vi "Main.vi"(7 "sweep rate, /min":dbl=0.2, 8 "sweep to:":dbl=-0.5, 9 "sweep":T6(radio)=enum."time_sweep") -> ()   [LabVIEW 2017] (continued)
                        n2125 = property on="data_caption" class="Str"() -> ("Value"=w2775:string)  [unwired: 2 in, 2 out]
                        n2126 = local read "Data file:"() -> (w2776:path)
                        n2127 = Concatenate Strings(w2775, "\r") -> (w2777:string)
                        n2128 = Write to Text File(file (use dialog)=w2776, text=w2777) -> ()  [unwired: 2 in, 3 out]
                      }
                      frame True {
                        # "records the fist line into the both upa nd down data file\nwhen table index=0"
                        n2129 = property on="Table Index" class="DigNum (strict)"() -> ("Value"=w2779:dbl)  [unwired: 2 in, 2 out]
                        n2130 = Equal To 0?(x=w2779) -> (x = 0?=w2778:bool)
                        n2131 = case shown="True" w2778 {
                          frame False {
                          }
                          frame True {
                            n2132 = property on="data_caption" class="Str"() -> ("Value"=w2783:string)  [unwired: 2 in, 2 out]
                            n2133 = local read "Data file:"() -> (w2780:path)
                            n2134 = Concatenate Strings(w2783, "\r") -> (w2782:string)
                            n2135 = Write to Text File(file (use dialog)=w2780, text=w2782) -> ()  [unwired: 2 in, 3 out]
                          }
                        }
                      }
                    }
                  }
                  frame True {
                    # "records the fist line into the both upa nd down data file\nwhen table index=0"
                    n2136 = property on="Table Index" class="DigNum (strict)"() -> ("Value"=w2787:dbl)  [unwired: 2 in, 2 out]
                    n2137 = property on="HyperLoop Index" class="DigNum (strict)"() -> ("Value"=w2788:dbl)  [unwired: 2 in, 2 out]
                    n2138 = Equal To 0?(x=w2787) -> (x = 0?=w2785:bool)
                    n2139 = Equal To 0?(x=w2788) -> (x = 0?=w2786:bool)
                    n2140 = And(x=w2786, y=w2785) -> (x .and. y?=w2784:bool)
                    n2141 = case shown="True" w2784 {
                      frame False {
                      }
                      frame True {
                        n2142 = property on="data_caption" class="Str"() -> ("Value"=w2792:string)  [unwired: 2 in, 2 out]
                        n2143 = local read "Data file:"() -> (w2789:path)
                        n2144 = Concatenate Strings(w2792, "\r") -> (w2791:string)
                        n2145 = Write to Text File(file (use dialog)=w2789, text=w2791) -> ()  [unwired: 2 in, 3 out]
                      }
                    }
                  }
                }
              }
            }
            n2146 = property on="Figure_axis" class="Arr (strict)"() -> ("Value"=w2759:string[])  [unwired: 2 in, 2 out]
            n2147 = property on="Xaxis" class="Ring (strict)"("Strings []"=w2759) -> ()  [unwired: 2 in, 2 out]
            n2148 = property on="Stop Sweep" class="Bool"("DisabledEnum"=T12."Enabled" ("Disabled")) -> ()  [unwired: 2 in, 2 out]
            n2149 = property on="Yright" class="Ring (strict)"("Strings []"=w2759) -> ()  [unwired: 2 in, 2 out]
            n2150 = property on="Yaxis" class="Ring (strict)"("Strings []"=w2759) -> ()  [unwired: 2 in, 2 out]
          }
        }
        n2151 = call "timeInSeconds.vi"() -> ("Numeric"=w1798:dbl)  [unwired: 2 in, 1 out]
        n2152 = while {
          shift-right: [w2844] -> _
          shift-left: w1797 -> [w2845]
          shift-right: [w2842] -> w1796
          shift-left: w1794 -> [w2841]
          tunnel: w1798 -> [w2839]
          stop <- w2832 stop-if-true
          # "initial value"
          # "Measure the selected channels"
          # "data array"
          # "this loop stops when target value is reached"
          # "error cluster to determine data flow"
          n2153 = stacked-sequence {
            tunnel: [_ _ w2866 _ _ _] -> w2833
            tunnel: [_ _ w2865 _ _ _] -> w2843
            tunnel: w2841 -> [_ _ w2859 _ _ _]
            tunnel: [w2851 _ _ _ _ _] -> w2840
            tunnel: w2839 -> [_ _ _ w2889 _ _]
            tunnel: [_ _ w2859 _ _ _] -> w2835
            tunnel: [_ _ _ _ _ w3552] -> w2831
            frame #0 {
              # "time is measured at the beginning\nand at the end of the cycle to\ncalculate delay time required to\nkeep set sweep rate"
              n2154 = flat-sequence {
                tunnel: [w2853] -> w2851
                frame #0 {
                  n2155 = property on="time delay, ms" class="DigNum (strict)"() -> ("Value"=w2852:dbl)  [unwired: 2 in, 2 out]
                  n2156 = Wait (ms)(milliseconds to wait=w2852) -> ()  [unwired: 1 out]
                }
                frame #1 {
                  n2157 = Tick Count (ms)() -> (millisecond timer value=w2853:u32)
                }
              }
            }
            frame #1 {
              w2854 = dbl[] []  # Empty array for data
              # "clear data array before each measurement cycle"
              n2158 = property on="data" class="Arr (strict)"("Value"=w2854) -> ()  [unwired: 2 in, 2 out]
            }
            frame #2 {
              # "add next sweep value to the data array"
              n2159 = property on="data" class="Arr (strict)"() -> ("Value"=w2864:dbl[])  [unwired: 2 in, 2 out]
              n2160 = property on="Sweep B" class="Bool (strict)"() -> ("Value"=w2856:bool)  [unwired: 2 in, 2 out]
              n2161 = local read "sweep"() -> (w2862:T6)
              n2162 = Not(x=w2856) -> (.not. x?=w2855:bool)
              n2163 = Equal?(x=w2862, y=T19."Radio Selection 7" ("sweep")) -> (x = y?=w2858:bool)
              n2164 = And(x=w2858, y=w2855) -> (x .and. y?=w2857:bool)
              n2165 = case shown="False" w2857 {
                tunnel: [w2873 w2885] -> w2866
                tunnel: [w2867 w2884] -> w2865
                tunnel: w2859 -> [_ w2882]
                tunnel: [w2867 w2882] -> w2860
                frame True {
                  n2166 = disable-structure shown="Disabled" {
                    disable-tunnel: [w2876 _] -> _
                    disable-tunnel: [w2875 _] -> _
                    frame Disabled {
                      n2167 = stacked-sequence {
                        tunnel: [_ w2878 _] -> w2876
                        tunnel: [_ _ w2880] -> w2875
                        frame #0 {
                          n2168 = local read "Hulk_SMS_addr"() -> (w2877:refnum<visa-resource-name>)
                          n2169 = VISA Clear(VISA resource name=w2877) -> ()  [unwired: 1 in, 2 out]
                        }
                        frame #1 {
                          # "acquires current output value"
                          n2170 = local read "Hulk_SMS_addr"() -> (w2879:refnum<visa-resource-name>)
                          n2171 = call "SMS_GET_OUTPUT.vi"("Hulk_SMS_addr"=w2879) -> ("Numeric"=w2878:dbl)  [unwired: 1 in, 2 out]
                        }
                        frame #2 {
                          # "checks, wheter ramp was finished"
                          n2172 = local read "Hulk_SMS_addr"() -> (w2881:refnum<visa-resource-name>)
                          n2173 = call "SMS_RAMP_STATUS.vi"("Hulk_SMS_addr"=w2881) -> ("selection"=w2880:bool)  [unwired: 1 in, 2 out]
                        }
                      }
                    }
                    frame Enabled {
                    }
                  }
                  n2174 = property on="iPS_addr_sweep" class="VISAName"() -> ("Value"=w2869:refnum<visa-resource-name>)  [unwired: 2 in, 2 out]
                  n2175 = property on="sweep to:" class="DigNum (strict)"() -> ("Value"=w2874:dbl)  [unwired: 2 in, 2 out]
                  n2176 = call "iPSread.vi"("iPSreadCtrl"=iPSreadCtrl."MagnetField", "VISA resource name"=w2869) -> ("number"=w2867:dbl)  [unwired: 6 in, 3 out]
                  n2177 = property on="Tolerance_Sweep" class="DigNum (strict)"() -> ("Value"=w2870:dbl)  [unwired: 2 in, 2 out]
                  n2178 = Subtract(x=w2867, y=w2874) -> (x-y=w2872:dbl)
                  n2179 = Absolute Value(x=w2872) -> (abs(x)=w2871:dbl)
                  n2180 = Less Or Equal?(x=w2871, y=w2870) -> (x <= y?=w2873:bool)
                }
                frame False {
                  # "calculate next value"
                  n2181 = call "CalculateNextValue.vi"("Target a 2"="sweep to:", "Channel a source value"=w2882, "Ch a sweep rate units/min"="sweep rate, /min", "time between points, sec"="time/point, sec", "Source a"=Source."Voltage") -> ("Target a"=w2884:dbl, "Boolean"=w2885:bool)
                }
              }
              n2182 = Build Array (concatenate)(w2864, w2860) -> (w2863:dbl[])
              n2183 = property on="data" class="Arr (strict)"("Value"=w2863) -> ()  [unwired: 2 in, 2 out]
            }
            frame #3 {
              n2184 = stacked-sequence "measurement sequence" {
                tunnel: w2889 -> [_ _ _ _ _ _ _ _ _ _ _ _ _ _ _ _ _ _ _ _ _ _ _ _ _ _ _ _ _ _ _ _ _ _ _ _ _ _ w3427 _ _ _ _ _ _ _ _ _ _ _ _ _]
                frame #0 {
                  # "check if in-phase\nsignal on lock-in 1 \nis to be measured"
                  n2185 = property on="data" class="Arr (strict)"() -> ("Value"=w2891:dbl[])  [unwired: 2 in, 2 out]
                  n2186 = local read "SR830 1 ip"() -> (w2890:bool)
                  n2187 = case shown="True" w2890 {
                    tunnel: w2891 -> [w2893 w2902]
                    tunnel: [w2893 w2901] -> w2892
                    frame False {
                      # "we are not measuring in phase signal on lock-in 1 (SR830_1_ip)"
                    }
                    frame True {
                      # "we are  measuring lock-in 1, in phase (SR830_1_ip)"
                      n2188 = local read "SR830 1 addr"() -> (w2895:u8)
                      n2189 = Number To Decimal String(number=w2895) -> (decimal integer string=w2894:string)  [unwired: 1 in]
                      n2190 = GPIB Write(0:w2894, 1:"OUTR?1") -> (6:w2900:errorcluster)  [unwired: 3 in, 1 out]
                      n2191 = GPIB Read(0:w2894, 1:3200, 3:w2900) -> (5:w2898:string)  [unwired: 2 in, 2 out]
                      n2192 = Fract/Exp String To Number(string=w2898) -> (number=w2897:dbl)  [unwired: 3 in, 1 out]
                      n2193 = Build Array (concatenate)(w2902, w2897) -> (w2901:dbl[])
                    }
                  }
                  n2194 = property on="data" class="Arr (strict)"("Value"=w2892) -> ()  [unwired: 2 in, 2 out]
                }
                frame #1 {
                  # "check if out-of-phase\nsignal on lock-in 1 \nis to be measured"
                  n2195 = property on="data" class="Arr (strict)"() -> ("Value"=w2904:dbl[])  [unwired: 2 in, 2 out]
                  n2196 = local read "SR830 1 oop"() -> (w2903:bool)
                  n2197 = case shown="True" w2903 {
                    tunnel: w2904 -> [w2906 w2915]
                    tunnel: [w2906 w2914] -> w2905
                    frame False {
                      # "we are not measuring out of phase signal on lock-in 1 (SR830_1_oop)"
                    }
                    frame True {
                      # "we are  measuring lock-in 1, out of phase (SR830_1_oop)"
                      n2198 = local read "SR830 1 addr"() -> (w2908:u8)
                      n2199 = Number To Decimal String(number=w2908) -> (decimal integer string=w2907:string)  [unwired: 1 in]
                      n2200 = GPIB Write(0:w2907, 1:"OUTR?2") -> (6:w2913:errorcluster)  [unwired: 3 in, 1 out]
                      n2201 = GPIB Read(0:w2907, 1:3200, 3:w2913) -> (5:w2911:string)  [unwired: 2 in, 2 out]
                      n2202 = Fract/Exp String To Number(string=w2911) -> (number=w2910:dbl)  [unwired: 3 in, 1 out]
                      n2203 = Build Array (concatenate)(w2915, w2910) -> (w2914:dbl[])
                    }
                  }
                  n2204 = property on="data" class="Arr (strict)"("Value"=w2905) -> ()  [unwired: 2 in, 2 out]
                }
                frame #2 {
                  # "check if in-phase\nsignal on lock-in 2 \nis to be measured"
                  n2205 = property on="data" class="Arr (strict)"() -> ("Value"=w2917:dbl[])  [unwired: 2 in, 2 out]
                  n2206 = local read "SR830 2 ip"() -> (w2916:bool)
                  n2207 = case shown="True" w2916 {
                    tunnel: w2917 -> [w2919 w2928]
                    tunnel: [w2919 w2927] -> w2918
                    frame False {
                      # "we are not measuring in phase signal on lock-in 2 (SR830_2_ip)"
                    }
                    frame True {
                      # "we are  measuring lock-in 2, in phase (SR830_2_ip)"
                      n2208 = local read "SR830 2 addr"() -> (w2921:u8)
                      n2209 = Number To Decimal String(number=w2921) -> (decimal integer string=w2920:string)  [unwired: 1 in]
                      n2210 = GPIB Write(0:w2920, 1:"OUTP?1") -> (6:w2926:errorcluster)  [unwired: 3 in, 1 out]
                      n2211 = GPIB Read(0:w2920, 1:3200, 3:w2926) -> (5:w2924:string)  [unwired: 2 in, 2 out]
                      n2212 = Fract/Exp String To Number(string=w2924) -> (number=w2923:dbl)  [unwired: 3 in, 1 out]
                      n2213 = Build Array (concatenate)(w2928, w2923) -> (w2927:dbl[])
                    }
                  }
                  n2214 = property on="data" class="Arr (strict)"("Value"=w2918) -> ()  [unwired: 2 in, 2 out]
                }
                frame #3 {
                  # "check if out-of-phase\nsignal on lock-in 2 \nis to be measured"
                  n2215 = property on="data" class="Arr (strict)"() -> ("Value"=w2930:dbl[])  [unwired: 2 in, 2 out]
                  n2216 = local read "SR830 2 oop"() -> (w2929:bool)
                  n2217 = case shown="True" w2929 {
                    tunnel: w2930 -> [w2932 w2941]
                    tunnel: [w2932 w2940] -> w2931
                    frame False {
                      # "we are not measuring out of phase signal on lock-in 2 (SR830_2_oop)"
                    }
                    frame True {
                      # "we are  measuring lock-in 2, out of phase (SR830_2_oop)"
                      n2218 = local read "SR830 2 addr"() -> (w2934:u8)
                      n2219 = Number To Decimal String(number=w2934) -> (decimal integer string=w2933:string)  [unwired: 1 in]
                      n2220 = GPIB Write(0:w2933, 1:"OUTP?2") -> (6:w2939:errorcluster)  [unwired: 3 in, 1 out]
                      n2221 = GPIB Read(0:w2933, 1:3200, 3:w2939) -> (5:w2937:string)  [unwired: 2 in, 2 out]
                      n2222 = Fract/Exp String To Number(string=w2937) -> (number=w2936:dbl)  [unwired: 3 in, 1 out]
                      n2223 = Build Array (concatenate)(w2941, w2936) -> (w2940:dbl[])
                    }
                  }
                  n2224 = property on="data" class="Arr (strict)"("Value"=w2931) -> ()  [unwired: 2 in, 2 out]
                }
                frame #4 {
                  # "check if in-phase\nsignal on lock-in 3 \nis to be measured"
                  n2225 = property on="data" class="Arr (strict)"() -> ("Value"=w2943:dbl[])  [unwired: 2 in, 2 out]
                  n2226 = local read "SR830 3 ip"() -> (w2942:bool)
                  n2227 = case shown="True" w2942 {
                    tunnel: w2943 -> [w2945 w2954]
                    tunnel: [w2945 w2953] -> w2944
                    frame False {
                      # "we are not measuring in phase signal on lock-in 3 (SR830_3_ip)"
                    }
                    frame True {
                      # "we are  measuring lock-in 3, in phase (SR830_3_ip)"
                      n2228 = local read "SR830 3 addr"() -> (w2947:u8)
                      n2229 = Number To Decimal String(number=w2947) -> (decimal integer string=w2946:string)  [unwired: 1 in]
                      n2230 = GPIB Write(0:w2946, 1:"OUTP?1") -> (6:w2952:errorcluster)  [unwired: 3 in, 1 out]
                      n2231 = GPIB Read(0:w2946, 1:3200, 3:w2952) -> (5:w2950:string)  [unwired: 2 in, 2 out]
                      n2232 = Fract/Exp String To Number(string=w2950) -> (number=w2949:dbl)  [unwired: 3 in, 1 out]
                      n2233 = Build Array (concatenate)(w2954, w2949) -> (w2953:dbl[])
                    }
                  }
                  n2234 = property on="data" class="Arr (strict)"("Value"=w2944) -> ()  [unwired: 2 in, 2 out]
                }
                frame #5 {
                  # "check if out-of-phase\nsignal on lock-in 3 \nis to be measured"
                  n2235 = property on="data" class="Arr (strict)"() -> ("Value"=w2956:dbl[])  [unwired: 2 in, 2 out]
                  n2236 = local read "SR830 3 oop"() -> (w2955:bool)
                  n2237 = case shown="True" w2955 {
                    tunnel: w2956 -> [w2958 w2967]
                    tunnel: [w2958 w2966] -> w2957
                    frame False {
                      # "we are not measuring out of phase signal on lock-in 3 (SR830_3_oop)"
                    }
                    frame True {
                      # "we are  measuring lock-in 3, out of phase (SR830_3_oop)"
                      n2238 = local read "SR830 3 addr"() -> (w2960:u8)
                      n2239 = Number To Decimal String(number=w2960) -> (decimal integer string=w2959:string)  [unwired: 1 in]
                      n2240 = GPIB Write(0:w2959, 1:"OUTP?2") -> (6:w2965:errorcluster)  [unwired: 3 in, 1 out]
                      n2241 = GPIB Read(0:w2959, 1:3200, 3:w2965) -> (5:w2963:string)  [unwired: 2 in, 2 out]
                      n2242 = Fract/Exp String To Number(string=w2963) -> (number=w2962:dbl)  [unwired: 3 in, 1 out]
                      n2243 = Build Array (concatenate)(w2967, w2962) -> (w2966:dbl[])
                    }
                  }
                  n2244 = property on="data" class="Arr (strict)"("Value"=w2957) -> ()  [unwired: 2 in, 2 out]
                }
                frame #6 {
                  # "check if in-phase\nsignal on lock-in 4 \nis to be measured"
                  n2245 = property on="data" class="Arr (strict)"() -> ("Value"=w2969:dbl[])  [unwired: 2 in, 2 out]
                  n2246 = local read "SR830 4 ip"() -> (w2968:bool)
                  n2247 = case shown="True" w2968 {
                    tunnel: w2969 -> [w2971 w2980]
                    tunnel: [w2971 w2979] -> w2970
                    frame False {
                      # "we are not measuring in phase signal on lock-in 4 (SR830_4_ip)"
                    }
                    frame True {
                      # "we are  measuring lock-in 4, in phase (SR830_4_ip)"
                      n2248 = local read "SR830 4 addr"() -> (w2973:u8)
                      n2249 = Number To Decimal String(number=w2973) -> (decimal integer string=w2972:string)  [unwired: 1 in]
                      n2250 = GPIB Write(0:w2972, 1:"OUTP?1") -> (6:w2978:errorcluster)  [unwired: 3 in, 1 out]
                      n2251 = GPIB Read(0:w2972, 1:3200, 3:w2978) -> (5:w2976:string)  [unwired: 2 in, 2 out]
                      n2252 = Fract/Exp String To Number(string=w2976) -> (number=w2975:dbl)  [unwired: 3 in, 1 out]
                      n2253 = Build Array (concatenate)(w2980, w2975) -> (w2979:dbl[])
                    }
                  }
                  n2254 = property on="data" class="Arr (strict)"("Value"=w2970) -> ()  [unwired: 2 in, 2 out]
                }
                frame #7 {
                  # "check if out-of-phase\nsignal on lock-in 4 \nis to be measured"
                  n2255 = property on="data" class="Arr (strict)"() -> ("Value"=w2982:dbl[])  [unwired: 2 in, 2 out]
                  n2256 = local read "SR830 4 oop"() -> (w2981:bool)
                  n2257 = case shown="True" w2981 {
                    tunnel: w2982 -> [w2984 w2993]
                    tunnel: [w2984 w2992] -> w2983
                    frame False {
                      # "we are not measuring out of phase signal on lock-in 4 (SR830_4_oop)"
                    }
                    frame True {
                      # "we are  measuring lock-in 4, out of phase (SR830_4_oop)"
                      n2258 = local read "SR830 4 addr"() -> (w2986:u8)
                      n2259 = Number To Decimal String(number=w2986) -> (decimal integer string=w2985:string)  [unwired: 1 in]
                      n2260 = GPIB Write(0:w2985, 1:"OUTP?2") -> (6:w2991:errorcluster)  [unwired: 3 in, 1 out]
                      n2261 = GPIB Read(0:w2985, 1:3200, 3:w2991) -> (5:w2989:string)  [unwired: 2 in, 2 out]
                      n2262 = Fract/Exp String To Number(string=w2989) -> (number=w2988:dbl)  [unwired: 3 in, 1 out]
                      n2263 = Build Array (concatenate)(w2993, w2988) -> (w2992:dbl[])
                    }
                  }
                  n2264 = property on="data" class="Arr (strict)"("Value"=w2983) -> ()  [unwired: 2 in, 2 out]
                }
                frame #8 {
                  # "check if in-phase\nsignal on lock-in 5 \nis to be measured"
                  n2265 = property on="data" class="Arr (strict)"() -> ("Value"=w2995:dbl[])  [unwired: 2 in, 2 out]
                  n2266 = local read "SR830 5 ip"() -> (w2994:bool)
                  n2267 = case shown="True" w2994 {
                    tunnel: w2995 -> [w2997 w3006]
                    tunnel: [w2997 w3005] -> w2996
                    frame False {
                      # "we are not measuring in phase signal on lock-in 5 (SR830_5_ip)"
                    }
                    frame True {
                      # "we are  measuring lock-in 5 in phase (SR830_5_ip)"
                      n2268 = local read "SR830 5 addr"() -> (w2999:u8)
                      n2269 = Number To Decimal String(number=w2999) -> (decimal integer string=w2998:string)  [unwired: 1 in]
                      n2270 = GPIB Write(0:w2998, 1:"OUTP?1") -> (6:w3004:errorcluster)  [unwired: 3 in, 1 out]
                      n2271 = GPIB Read(0:w2998, 1:3200, 3:w3004) -> (5:w3002:string)  [unwired: 2 in, 2 out]
                      n2272 = Fract/Exp String To Number(string=w3002) -> (number=w3001:dbl)  [unwired: 3 in, 1 out]
                      n2273 = Build Array (concatenate)(w3006, w3001) -> (w3005:dbl[])
                    }
                  }
                  n2274 = property on="data" class="Arr (strict)"("Value"=w2996) -> ()  [unwired: 2 in, 2 out]
                }
                frame #9 {
                  # "check if out-of-phase\nsignal on lock-in 5 \nis to be measured"
                  n2275 = property on="data" class="Arr (strict)"() -> ("Value"=w3008:dbl[])  [unwired: 2 in, 2 out]
                  n2276 = local read "SR830 5 oop"() -> (w3007:bool)
                  n2277 = case shown="True" w3007 {
                    tunnel: w3008 -> [w3010 w3019]
                    tunnel: [w3010 w3018] -> w3009
                    frame False {
                      # "we are not measuring out of phase signal on lock-in 5 (SR830_5_oop)"
                    }
                    frame True {
                      # "we are  measuring lock-in 5 out of phase (SR830_5_oop)"
                      n2278 = local read "SR830 5 addr"() -> (w3012:u8)
                      n2279 = Number To Decimal String(number=w3012) -> (decimal integer string=w3011:string)  [unwired: 1 in]
                      n2280 = GPIB Write(0:w3011, 1:"OUTP?2") -> (6:w3017:errorcluster)  [unwired: 3 in, 1 out]
                      n2281 = GPIB Read(0:w3011, 1:3200, 3:w3017) -> (5:w3015:string)  [unwired: 2 in, 2 out]
                      n2282 = Fract/Exp String To Number(string=w3015) -> (number=w3014:dbl)  [unwired: 3 in, 1 out]
                      n2283 = Build Array (concatenate)(w3019, w3014) -> (w3018:dbl[])
                    }
                  }
                  n2284 = property on="data" class="Arr (strict)"("Value"=w3009) -> ()  [unwired: 2 in, 2 out]
                }
                frame #10 {
                  # "check if in-phase\nsignal on lock-in 6 \nis to be measured"
                  n2285 = property on="data" class="Arr (strict)"() -> ("Value"=w3021:dbl[])  [unwired: 2 in, 2 out]
                  n2286 = local read "SR830_6_ip"() -> (w3020:bool)
                  n2287 = case shown="True" w3020 {
                    tunnel: w3021 -> [w3023 w3032]
                    tunnel: [w3023 w3031] -> w3022
                    frame False {
                      # "we are not measuring in phase signal on lock-in 6 (SR830_6_ip)"
                    }
                    frame True {
                      # "we are  measuring lock-in 6 in phase (SR830_6_ip)"
                      n2288 = local read "SR830_6"() -> (w3025:u8)
                      n2289 = Number To Decimal String(number=w3025) -> (decimal integer string=w3024:string)  [unwired: 1 in]
                      n2290 = GPIB Write(0:w3024, 1:"OUTR?1") -> (6:w3030:errorcluster)  [unwired: 3 in, 1 out]
                      n2291 = GPIB Read(0:w3024, 1:3200, 3:w3030) -> (5:w3028:string)  [unwired: 2 in, 2 out]
                      n2292 = Fract/Exp String To Number(string=w3028) -> (number=w3027:dbl)  [unwired: 3 in, 1 out]
                      n2293 = Build Array (concatenate)(w3032, w3027) -> (w3031:dbl[])
                    }
                  }
                  n2294 = property on="data" class="Arr (strict)"("Value"=w3022) -> ()  [unwired: 2 in, 2 out]
                }
                frame #11 {
                  # "check if out-of-phase\nsignal on lock-in 6 \nis to be measured"
                  n2295 = property on="data" class="Arr (strict)"() -> ("Value"=w3034:dbl[])  [unwired: 2 in, 2 out]
                  n2296 = local read "SR830_6_oop"() -> (w3033:bool)
                  n2297 = case shown="True" w3033 {
                    tunnel: w3034 -> [w3036 w3045]
                    tunnel: [w3036 w3044] -> w3035
                    frame False {
                      # "we are not measuring out of phase signal on lock-in 6 (SR830_6_oop)"
                    }
                    frame True {
                      # "we are  measuring lock-in 6, out of phase (SR830_6_oop)"
                      n2298 = local read "SR830_6"() -> (w3038:u8)
                      n2299 = Number To Decimal String(number=w3038) -> (decimal integer string=w3037:string)  [unwired: 1 in]
                      n2300 = GPIB Write(0:w3037, 1:"OUTR?2") -> (6:w3043:errorcluster)  [unwired: 3 in, 1 out]
                      n2301 = GPIB Read(0:w3037, 1:3200, 3:w3043) -> (5:w3041:string)  [unwired: 2 in, 2 out]
                      n2302 = Fract/Exp String To Number(string=w3041) -> (number=w3040:dbl)  [unwired: 3 in, 1 out]
                      n2303 = Build Array (concatenate)(w3045, w3040) -> (w3044:dbl[])
                    }
                  }
                  n2304 = property on="data" class="Arr (strict)"("Value"=w3035) -> ()  [unwired: 2 in, 2 out]
                }
                frame #12 {
                  # "check if in-phase\nsignal on lock-in 7 \nis to be measured"
                  n2305 = property on="data" class="Arr (strict)"() -> ("Value"=w3047:dbl[])  [unwired: 2 in, 2 out]
                  n2306 = local read "SR830_7_ip"() -> (w3046:bool)
                  n2307 = case shown="True" w3046 {
                    tunnel: w3047 -> [w3049 w3058]
                    tunnel: [w3049 w3057] -> w3048
                    frame False {
                    }
                    frame True {
                      # "we are  measuring lock-in 7 in phase (SR830_7_ip)"
                      n2308 = local read "SR830_7"() -> (w3051:u8)
                      n2309 = Number To Decimal String(number=w3051) -> (decimal integer string=w3050:string)  [unwired: 1 in]
                      n2310 = GPIB Write(0:w3050, 1:"OUTR?1") -> (6:w3056:errorcluster)  [unwired: 3 in, 1 out]
                      n2311 = GPIB Read(0:w3050, 1:3200, 3:w3056) -> (5:w3054:string)  [unwired: 2 in, 2 out]
                      n2312 = Fract/Exp String To Number(string=w3054) -> (number=w3053:dbl)  [unwired: 3 in, 1 out]
                      n2313 = Build Array (concatenate)(w3058, w3053) -> (w3057:dbl[])
                    }
                  }
                  n2314 = property on="data" class="Arr (strict)"("Value"=w3048) -> ()  [unwired: 2 in, 2 out]
                }
                frame #13 {
                  # "check if out-of-phase\nsignal on lock-in 7 \nis to be measured"
                  n2315 = property on="data" class="Arr (strict)"() -> ("Value"=w3060:dbl[])  [unwired: 2 in, 2 out]
                  n2316 = local read "SR830_7_oop"() -> (w3059:bool)
                  n2317 = case shown="True" w3059 {
                    tunnel: w3060 -> [w3062 w3071]
                    tunnel: [w3062 w3070] -> w3061
                    frame False {
                    }
                    frame True {
                      # "we are  measuring lock-in 7 out of phase (SR830_7_oop)"
                      n2318 = local read "SR830_7"() -> (w3064:u8)
                      n2319 = Number To Decimal String(number=w3064) -> (decimal integer string=w3063:string)  [unwired: 1 in]
                      n2320 = GPIB Write(0:w3063, 1:"OUTR?2") -> (6:w3069:errorcluster)  [unwired: 3 in, 1 out]
                      n2321 = GPIB Read(0:w3063, 1:3200, 3:w3069) -> (5:w3067:string)  [unwired: 2 in, 2 out]
                      n2322 = Fract/Exp String To Number(string=w3067) -> (number=w3066:dbl)  [unwired: 3 in, 1 out]
                      n2323 = Build Array (concatenate)(w3071, w3066) -> (w3070:dbl[])
                    }
                  }
                  n2324 = property on="data" class="Arr (strict)"("Value"=w3061) -> ()  [unwired: 2 in, 2 out]
                }
                frame #14 {
                  # "check if in-phase\nsignal on lock-in 8 \nis to be measured"
                  n2325 = property on="data" class="Arr (strict)"() -> ("Value"=w3073:dbl[])  [unwired: 2 in, 2 out]
                  n2326 = local read "SR830_8_ip"() -> (w3072:bool)
                  n2327 = case shown="True" w3072 {
                    tunnel: w3073 -> [w3075 w3084]
                    tunnel: [w3075 w3083] -> w3074
                    frame False {
                    }
                    frame True {
                      # "we are  measuring lock-in 8 in phase (SR830_8_ip)"
                      n2328 = local read "SR830_8"() -> (w3077:u8)
                      n2329 = Number To Decimal String(number=w3077) -> (decimal integer string=w3076:string)  [unwired: 1 in]
                      n2330 = GPIB Write(0:w3076, 1:"OUTR?1") -> (6:w3082:errorcluster)  [unwired: 3 in, 1 out]
                      n2331 = GPIB Read(0:w3076, 1:3200, 3:w3082) -> (5:w3080:string)  [unwired: 2 in, 2 out]
                      n2332 = Fract/Exp String To Number(string=w3080) -> (number=w3079:dbl)  [unwired: 3 in, 1 out]
                      n2333 = Build Array (concatenate)(w3084, w3079) -> (w3083:dbl[])
                    }
                  }
                  n2334 = property on="data" class="Arr (strict)"("Value"=w3074) -> ()  [unwired: 2 in, 2 out]
                }
                frame #15 {
                  # "check if out-of-phase\nsignal on lock-in 8 \nis to be measured"
                  n2335 = property on="data" class="Arr (strict)"() -> ("Value"=w3086:dbl[])  [unwired: 2 in, 2 out]
                  n2336 = local read "SR830_8_oop"() -> (w3085:bool)
                  n2337 = case shown="True" w3085 {
                    tunnel: w3086 -> [w3088 w3097]
                    tunnel: [w3088 w3096] -> w3087
                    frame False {
                    }
                    frame True {
                      # "we are  measuring lock-in 8 out of phase (SR830_8_oop)"
                      n2338 = local read "SR830_8"() -> (w3090:u8)
                      n2339 = Number To Decimal String(number=w3090) -> (decimal integer string=w3089:string)  [unwired: 1 in]
                      n2340 = GPIB Write(0:w3089, 1:"OUTR?2") -> (6:w3095:errorcluster)  [unwired: 3 in, 1 out]
                      n2341 = GPIB Read(0:w3089, 1:3200, 3:w3095) -> (5:w3093:string)  [unwired: 2 in, 2 out]
                      n2342 = Fract/Exp String To Number(string=w3093) -> (number=w3092:dbl)  [unwired: 3 in, 1 out]
                      n2343 = Build Array (concatenate)(w3097, w3092) -> (w3096:dbl[])
                    }
                  }
                  n2344 = property on="data" class="Arr (strict)"("Value"=w3087) -> ()  [unwired: 2 in, 2 out]
                }
                frame #16 {
                  # "Measure MFLI_V if \nit is checked"
                  n2345 = property on="MFLI_V1" class="Bool (strict)"() -> ("Value"=w3098:bool)  [unwired: 2 in, 2 out]
                  n2346 = property on="data" class="Arr (strict)"() -> ("Value"=w3100:dbl[])  [unwired: 2 in, 2 out]
                  n2347 = case shown="True" w3098 {
                    tunnel: w3100 -> [w3101 w3106]
                    tunnel: [w3101 w3105] -> w3099
                    frame False {
                      # "We are not recording Step Value if it is linetrace"
                    }
                    frame True {
                      n2348 = flat-sequence {
                        tunnel: [w3110] -> w3104
                        tunnel: [w3109] -> w3103
                        tunnel: [w3108] -> w3102
                        frame #0 {
                          n2349 = property on="HandleOut" class="Clust (strict)"() -> ("Value"=w3112:T5)  [unwired: 2 in, 2 out]
                          n2350 = call "MFLIcontrol.vi"("MFLI function"=MFLIcommand."measure XY on demod0", "handle in"=w3112) -> ("Demod Sample Out 2"=w3107:T22)  [unwired: 6 in, 3 out]
                          n2351 = Unbundle(w3107) -> ("X (Vrms)"=w3110:dbl, "Y (Vrms)"=w3109:dbl, "Freq (Hz)"=w3108:dbl)  [unwired: 6 out]
                        }
                      }
                      n2352 = Build Array (concatenate)(w3106, w3104, w3103, w3102) -> (w3105:dbl[])
                    }
                  }
                  n2353 = property on="data" class="Arr (strict)"("Value"=w3099) -> ()  [unwired: 2 in, 2 out]
                }
                frame #17 {
                  # "Measure MFLI_I if \nit is checked"
                  n2354 = property on="MFLI_I1" class="Bool (strict)"() -> ("Value"=w3113:bool)  [unwired: 2 in, 2 out]
                  n2355 = property on="data" class="Arr (strict)"() -> ("Value"=w3115:dbl[])  [unwired: 2 in, 2 out]
                  n2356 = case shown="True" w3113 {
                    tunnel: w3115 -> [w3116 w3121]
                    tunnel: [w3116 w3120] -> w3114
                    frame False {
                      # "We are not recording Step Value if it is linetrace"
                    }
                    frame True {
                      n2357 = flat-sequence {
                        tunnel: [w3124] -> w3119
                        tunnel: [w3123] -> w3118
                        tunnel: [w3122] -> w3117
                        frame #0 {
                          n2358 = property on="HandleOut" class="Clust (strict)"() -> ("Value"=w3127:T5)  [unwired: 2 in, 2 out]
                          n2359 = call "MFLIcontrol.vi"("MFLI function"=MFLIcommand."measure current", "handle in"=w3127) -> ("Demod Sample Out 3"=w3125:T22)  [unwired: 6 in, 3 out]
                          n2360 = Unbundle(w3125) -> ("X (Vrms)"=w3124:dbl, "Y (Vrms)"=w3123:dbl, "Freq (Hz)"=w3122:dbl)  [unwired: 6 out]
                        }
                      }
                      n2361 = Build Array (concatenate)(w3121, w3119, w3118, w3117) -> (w3120:dbl[])
                    }
                  }
                  n2362 = property on="data" class="Arr (strict)"("Value"=w3114) -> ()  [unwired: 2 in, 2 out]
                }
                frame #18 {
                  # "Measure MFLI_V if \nit is checked"
                  n2363 = local read "MFLI_V2"() -> (w3128:bool)
                  n2364 = property on="data" class="Arr (strict)"() -> ("Value"=w3130:dbl[])  [unwired: 2 in, 2 out]
                  n2365 = case shown="True" w3128 {
                    tunnel: w3130 -> [w3131 w3136]
                    tunnel: [w3131 w3135] -> w3129
                    frame False {
                    }
                    frame True {
                      n2366 = flat-sequence {
                        tunnel: [w3141] -> w3134
                        tunnel: [w3140] -> w3133
                        tunnel: [w3139] -> w3132
                        frame #0 {
                          n2367 = property on="Handle Out 2" class="Clust (strict)"() -> ("Value"=w3137:T5)  [unwired: 2 in, 2 out]
                          n2368 = call "MFLIcontrol.vi"("MFLI function"=MFLIcommand."measure XY on demod0", "handle in"=w3137) -> ("Demod Sample Out 2"=w3138:T22)  [unwired: 6 in, 3 out]
                          n2369 = Unbundle(w3138) -> ("X (Vrms)"=w3141:dbl, "Y (Vrms)"=w3140:dbl, "Freq (Hz)"=w3139:dbl)  [unwired: 6 out]
                        }
                      }
                      n2370 = Build Array (concatenate)(w3136, w3134, w3133, w3132) -> (w3135:dbl[])
                    }
                  }
                  n2371 = property on="data" class="Arr (strict)"("Value"=w3129) -> ()  [unwired: 2 in, 2 out]
                }
                frame #19 {
                  # "Measure MFLI_I if \nit is checked"
                  n2372 = local read "MFLI_I2"() -> (w3143:bool)
                  n2373 = property on="data" class="Arr (strict)"() -> ("Value"=w3145:dbl[])  [unwired: 2 in, 2 out]
                  n2374 = case shown="True" w3143 {
                    tunnel: w3145 -> [w3146 w3151]
                    tunnel: [w3146 w3150] -> w3144
                    frame False {
                    }
                    frame True {
                      n2375 = flat-sequence {
                        tunnel: [w3156] -> w3149
                        tunnel: [w3155] -> w3148
                        tunnel: [w3154] -> w3147
                        frame #0 {
                          n2376 = property on="Handle Out 2" class="Clust (strict)"() -> ("Value"=w3153:T5)  [unwired: 2 in, 2 out]
                          n2377 = call "MFLIcontrol.vi"("MFLI function"=MFLIcommand."measure current", "handle in"=w3153) -> ("Demod Sample Out 3"=w3152:T22)  [unwired: 6 in, 3 out]
                          n2378 = Unbundle(w3152) -> ("X (Vrms)"=w3156:dbl, "Y (Vrms)"=w3155:dbl, "Freq (Hz)"=w3154:dbl)  [unwired: 6 out]
                        }
                      }
                      n2379 = Build Array (concatenate)(w3151, w3149, w3148, w3147) -> (w3150:dbl[])
                    }
                  }
                  n2380 = property on="data" class="Arr (strict)"("Value"=w3144) -> ()  [unwired: 2 in, 2 out]
                }
                frame #20 {
                  # "check if voltage \non 2400 SouceMeter 1\nis to be measured"
                  n2381 = property on="data" class="Arr (strict)"() -> ("Value"=w3159:dbl[])  [unwired: 2 in, 2 out]
                  n2382 = local read "2400 1 meas v"() -> (w3158:bool)
                  n2383 = case shown="True" w3158 {
                    tunnel: w3159 -> [w3161 w3172]
                    tunnel: [w3161 w3171] -> w3160
                    frame False {
                      # "we are not measuring 2400 1, voltage (2400_1_v)"
                    }
                    frame True {
                      # "we are  measuring 2400 1, voltage (2400_1_v)"
                      n2384 = local read "2400 1 addr"() -> (w3166:u8)
                      n2385 = Number To Decimal String(number=w3166) -> (decimal integer string=w3165:string)  [unwired: 1 in]
                      n2386 = GPIB Write(0:w3165, 1:":READ?") -> (6:w3170:errorcluster)  [unwired: 3 in, 1 out]
                      n2387 = GPIB Read(0:w3165, 1:3200, 3:w3170) -> (5:w3163:string)  [unwired: 2 in, 2 out]
                      n2388 = String Subset(string=w3163, length (rest)=13) -> (substring=w3162:string)  [unwired: 1 in]
                      n2389 = Fract/Exp String To Number(string=w3162) -> (number=w3168:dbl)  [unwired: 3 in, 1 out]
                      n2390 = Build Array (concatenate)(w3172, w3168) -> (w3171:dbl[])
                    }
                  }
                  n2391 = property on="data" class="Arr (strict)"("Value"=w3160) -> ()  [unwired: 2 in, 2 out]
                }
                frame #21 {
                  # "check if current \non 2400 SouceMeter 1\nis to be measured"
                  n2392 = property on="data" class="Arr (strict)"() -> ("Value"=w3174:dbl[])  [unwired: 2 in, 2 out]
                  n2393 = local read "2400 1 meas i"() -> (w3173:bool)
                  n2394 = case shown="True" w3173 {
                    tunnel: w3174 -> [w3176 w3188]
                    tunnel: [w3176 w3187] -> w3175
                    frame False {
                      # "we are not measuring 2400 1, current (2400_1_i)"
                    }
                    frame True {
                      # "we are  measuring 2400 1, current (2400_1_i)"
                      n2395 = local read "2400 1 addr"() -> (w3182:u8)
                      n2396 = Number To Decimal String(number=w3182) -> (decimal integer string=w3181:string)  [unwired: 1 in]
                      n2397 = GPIB Write(0:w3181, 1:":READ?") -> (6:w3186:errorcluster)  [unwired: 3 in, 1 out]
                      n2398 = GPIB Read(0:w3181, 1:3200, 3:w3186) -> (5:w3179:string)  [unwired: 2 in, 2 out]
                      n2399 = String Subset(string=w3179, offset (0)=14, length (rest)=13) -> (substring=w3178:string)
                      n2400 = Fract/Exp String To Number(string=w3178) -> (number=w3184:dbl)  [unwired: 3 in, 1 out]
                      n2401 = Build Array (concatenate)(w3188, w3184) -> (w3187:dbl[])
                    }
                  }
                  n2402 = property on="data" class="Arr (strict)"("Value"=w3175) -> ()  [unwired: 2 in, 2 out]
                }
                frame #22 {
                  # "check if voltage \non 2400 SouceMeter 2\nis to be measured"
                  n2403 = property on="data" class="Arr (strict)"() -> ("Value"=w3190:dbl[])  [unwired: 2 in, 2 out]
                  n2404 = local read "2400 2 meas v"() -> (w3189:bool)
                  n2405 = case shown="True" w3189 {
                    tunnel: w3190 -> [w3192 w3203]
                    tunnel: [w3192 w3202] -> w3191
                    frame False {
                      # "we are not measuring 2400 2, voltage (2400_2_v)"
                    }
                    frame True {
                      # "we are  measuring 2400 2, voltage (2400_2_v)"
                      n2406 = local read "2400 2 addr"() -> (w3197:u8)
                      n2407 = Number To Decimal String(number=w3197) -> (decimal integer string=w3196:string)  [unwired: 1 in]
                      n2408 = GPIB Write(0:w3196, 1:":READ?") -> (6:w3201:errorcluster)  [unwired: 3 in, 1 out]
                      n2409 = GPIB Read(0:w3196, 1:3200, 3:w3201) -> (5:w3194:string)  [unwired: 2 in, 2 out]
                      n2410 = String Subset(string=w3194, length (rest)=13) -> (substring=w3193:string)  [unwired: 1 in]
                      n2411 = Fract/Exp String To Number(string=w3193) -> (number=w3199:dbl)  [unwired: 3 in, 1 out]
                      n2412 = Build Array (concatenate)(w3203, w3199) -> (w3202:dbl[])
                    }
                  }
                  n2413 = property on="data" class="Arr (strict)"("Value"=w3191) -> ()  [unwired: 2 in, 2 out]
                }
                frame #23 {
                  # "check if current \non 2400 SouceMeter 2\nis to be measured"
                  n2414 = property on="data" class="Arr (strict)"() -> ("Value"=w3205:dbl[])  [unwired: 2 in, 2 out]
                  n2415 = local read "2400 2 meas i"() -> (w3204:bool)
                  n2416 = case shown="True" w3204 {
                    tunnel: w3205 -> [w3207 w3219]
                    tunnel: [w3207 w3218] -> w3206
                    frame False {
                      # "we are not measuring 2400 2, current (2400_2_i)"
                    }
                    frame True {
                      # "we are  measuring 2400 2, current (2400_2_i)"
                      n2417 = local read "2400 2 addr"() -> (w3213:u8)
                      n2418 = Number To Decimal String(number=w3213) -> (decimal integer string=w3212:string)  [unwired: 1 in]
                      n2419 = GPIB Write(0:w3212, 1:":READ?") -> (6:w3217:errorcluster)  [unwired: 3 in, 1 out]
                      n2420 = GPIB Read(0:w3212, 1:3200, 3:w3217) -> (5:w3210:string)  [unwired: 2 in, 2 out]
                      n2421 = String Subset(string=w3210, offset (0)=14, length (rest)=13) -> (substring=w3209:string)
                      n2422 = Fract/Exp String To Number(string=w3209) -> (number=w3215:dbl)  [unwired: 3 in, 1 out]
                      n2423 = Build Array (concatenate)(w3219, w3215) -> (w3218:dbl[])
                    }
                  }
                  n2424 = property on="data" class="Arr (strict)"("Value"=w3206) -> ()  [unwired: 2 in, 2 out]
                }
                frame #24 {
                  # "check if voltage \non 2400 SouceMeter 3\nis to be measured"
                  n2425 = property on="data" class="Arr (strict)"() -> ("Value"=w3221:dbl[])  [unwired: 2 in, 2 out]
                  n2426 = local read "2400 3 meas v"() -> (w3220:bool)
                  n2427 = case shown="True" w3220 {
                    tunnel: w3221 -> [w3223 w3234]
                    tunnel: [w3223 w3233] -> w3222
                    frame False {
                      # "we are not measuring 2400 3, voltage (2400_3_v)"
                    }
                    frame True {
                      # "we are  measuring 2400 3, voltage (2400_3_v)"
                      n2428 = local read "2400 3 addr"() -> (w3228:u8)
                      n2429 = Number To Decimal String(number=w3228) -> (decimal integer string=w3227:string)  [unwired: 1 in]
                      n2430 = GPIB Write(0:w3227, 1:":READ?") -> (6:w3232:errorcluster)  [unwired: 3 in, 1 out]
                      n2431 = GPIB Read(0:w3227, 1:3200, 3:w3232) -> (5:w3225:string)  [unwired: 2 in, 2 out]
                      n2432 = String Subset(string=w3225, length (rest)=13) -> (substring=w3224:string)  [unwired: 1 in]
                      n2433 = Fract/Exp String To Number(string=w3224) -> (number=w3230:dbl)  [unwired: 3 in, 1 out]
                      n2434 = Build Array (concatenate)(w3234, w3230) -> (w3233:dbl[])
                    }
                  }
                  n2435 = property on="data" class="Arr (strict)"("Value"=w3222) -> ()  [unwired: 2 in, 2 out]
                }
                frame #25 {
                  # "check if current \non 2400 SouceMeter 3\nis to be measured"
                  n2436 = property on="data" class="Arr (strict)"() -> ("Value"=w3236:dbl[])  [unwired: 2 in, 2 out]
                  n2437 = local read "2400 3 meas i"() -> (w3235:bool)
                  n2438 = case shown="True" w3235 {
                    tunnel: w3236 -> [w3238 w3250]
                    tunnel: [w3238 w3249] -> w3237
                    frame False {
                      # "we are not measuring 2400 3, current (2400_3_i)"
                    }
                    frame True {
                      # "we are  measuring 2400 3, current (2400_3_i)"
                      n2439 = local read "2400 3 addr"() -> (w3244:u8)
                      n2440 = Number To Decimal String(number=w3244) -> (decimal integer string=w3243:string)  [unwired: 1 in]
                      n2441 = GPIB Write(0:w3243, 1:":READ?") -> (6:w3248:errorcluster)  [unwired: 3 in, 1 out]
                      n2442 = GPIB Read(0:w3243, 1:3200, 3:w3248) -> (5:w3241:string)  [unwired: 2 in, 2 out]
                      n2443 = String Subset(string=w3241, offset (0)=14, length (rest)=13) -> (substring=w3240:string)
                      n2444 = Fract/Exp String To Number(string=w3240) -> (number=w3246:dbl)  [unwired: 3 in, 1 out]
                      n2445 = Build Array (concatenate)(w3250, w3246) -> (w3249:dbl[])
                    }
                  }
                  n2446 = property on="data" class="Arr (strict)"("Value"=w3237) -> ()  [unwired: 2 in, 2 out]
                }
                frame #26 {
                  # "check if 1st channel \non Keithley 2182A 1\nis to be measured"
                  n2447 = property on="data" class="Arr (strict)"() -> ("Value"=w3252:dbl[])  [unwired: 2 in, 2 out]
                  n2448 = local read "2182A 1 ch1"() -> (w3251:bool)
                  n2449 = case shown="True" w3251 {
                    tunnel: w3252 -> [w3254 w3263]
                    tunnel: [w3254 w3262] -> w3253
                    frame False {
                      # "we are not measuring 2182A 1 channel 1 (2182A_1_ch1)"
                    }
                    frame True {
                      # "we are  measuring 2182A 1 channel 1 (2182A_1_ch1)"
                      n2450 = local read "2182A 1 addr"() -> (w3257:u8)
                      n2451 = Number To Decimal String(number=w3257) -> (decimal integer string=w3256:string)  [unwired: 1 in]
                      n2452 = GPIB Write(0:w3256, 1:":SENSe:DATA:FRES?") -> (6:w3261:errorcluster)  [unwired: 3 in, 1 out]
                      n2453 = GPIB Read(0:w3256, 1:200, 3:w3261) -> (5:w3255:string)  [unwired: 2 in, 2 out]
                      n2454 = Fract/Exp String To Number(string=w3255) -> (number=w3259:dbl)  [unwired: 3 in, 1 out]
                      n2455 = Build Array (concatenate)(w3263, w3259) -> (w3262:dbl[])
                    }
                  }
                  n2456 = property on="data" class="Arr (strict)"("Value"=w3253) -> ()  [unwired: 2 in, 2 out]
                }
                frame #27 {
                  # "check if 2nd channel \non Keithley 2182A 1\nis to be measured"
                  n2457 = property on="data" class="Arr (strict)"() -> ("Value"=w3265:dbl[])  [unwired: 2 in, 2 out]
                  n2458 = local read "2182A 1 ch2"() -> (w3264:bool)
                  n2459 = case shown="True" w3264 {
                    tunnel: w3265 -> [w3267 w3280]
                    tunnel: [w3267 w3279] -> w3266
                    frame False {
                      # "we are not measuring 2182A 1 channel 2 (2182A_1_ch2)"
                    }
                    frame True {
                      # "switching to channel 2 and then\nback to channel 1"
                      # "we are  measuring 2182A 1 channel 2 (2182A_1_ch2)"
                      n2460 = local read "2182A 1 addr"() -> (w3274:u8)
                      n2461 = Number To Decimal String(number=w3274) -> (decimal integer string=w3269:string)  [unwired: 1 in]
                      n2462 = GPIB Write(0:w3269, 1:":SENSe:CHAN 2") -> (6:w3271:errorcluster)  [unwired: 3 in, 1 out]
                      n2463 = GPIB Write(0:w3269, 1:":SENSe:DATA:FRES?", 3:w3271) -> (6:w3278:errorcluster)  [unwired: 2 in, 1 out]
                      n2464 = GPIB Read(0:w3269, 1:200, 3:w3278) -> (5:w3273:string, 7:w3270:errorcluster)  [unwired: 2 in, 1 out]
                      n2465 = GPIB Write(0:w3269, 1:":SENSe:CHAN 1", 3:w3270) -> ()  [unwired: 2 in, 2 out]
                      n2466 = Fract/Exp String To Number(string=w3273) -> (number=w3276:dbl)  [unwired: 3 in, 1 out]
                      n2467 = Build Array (concatenate)(w3280, w3276) -> (w3279:dbl[])
                    }
                  }
                  n2468 = property on="data" class="Arr (strict)"("Value"=w3266) -> ()  [unwired: 2 in, 2 out]
                }
                frame #28 {
                  # "check if 1st channel \non Keithley 2182A 2\nis to be measured"
                  n2469 = property on="data" class="Arr (strict)"() -> ("Value"=w3282:dbl[])  [unwired: 2 in, 2 out]
                  n2470 = local read "2182A 2 ch1"() -> (w3281:bool)
                  n2471 = case shown="True" w3281 {
                    tunnel: w3282 -> [w3284 w3293]
                    tunnel: [w3284 w3292] -> w3283
                    frame False {
                      # "we are not measuring 2182A 2 channel 1 (2182A_2_ch1)"
                    }
                    frame True {
                      # "we are  measuring 2182A 2 channel 1 (2182A_2_ch1)"
                      n2472 = local read "2182A 2 addr"() -> (w3287:u8)
                      n2473 = Number To Decimal String(number=w3287) -> (decimal integer string=w3286:string)  [unwired: 1 in]
                      n2474 = GPIB Write(0:w3286, 1:":SENSe:DATA:FRES?") -> (6:w3291:errorcluster)  [unwired: 3 in, 1 out]
                      n2475 = GPIB Read(0:w3286, 1:200, 3:w3291) -> (5:w3285:string)  [unwired: 2 in, 2 out]
                      n2476 = Fract/Exp String To Number(string=w3285) -> (number=w3289:dbl)  [unwired: 3 in, 1 out]
                      n2477 = Build Array (concatenate)(w3293, w3289) -> (w3292:dbl[])
                    }
                  }
                  n2478 = property on="data" class="Arr (strict)"("Value"=w3283) -> ()  [unwired: 2 in, 2 out]
                }
                frame #29 {
                  # "check if 2nd channel \non Keithley 2182A 2\nis to be measured"
                  n2479 = property on="data" class="Arr (strict)"() -> ("Value"=w3295:dbl[])  [unwired: 2 in, 2 out]
                  n2480 = local read "2182A 2 ch2"() -> (w3294:bool)
                  n2481 = case shown="True" w3294 {
                    tunnel: w3295 -> [w3297 w3310]
                    tunnel: [w3297 w3309] -> w3296
                    frame False {
                      # "we are not measuring 2182A 2 channel 2 (2182A_2_ch2)"
                    }
                    frame True {
                      # "switching to channel 2 and then\nback to channel 1"
                      # "we are  measuring 2182A 2 channel 2 (2182A_2_ch2)"
                      n2482 = local read "2182A 2 addr"() -> (w3304:u8)
                      n2483 = Number To Decimal String(number=w3304) -> (decimal integer string=w3299:string)  [unwired: 1 in]
                      n2484 = GPIB Write(0:w3299, 1:":SENSe:CHAN 2") -> (6:w3301:errorcluster)  [unwired: 3 in, 1 out]
                      n2485 = GPIB Write(0:w3299, 1:":SENSe:DATA:FRES?", 3:w3301) -> (6:w3308:errorcluster)  [unwired: 2 in, 1 out]
                      n2486 = GPIB Read(0:w3299, 1:200, 3:w3308) -> (5:w3303:string, 7:w3300:errorcluster)  [unwired: 2 in, 1 out]
                      n2487 = GPIB Write(0:w3299, 1:":SENSe:CHAN 1", 3:w3300) -> ()  [unwired: 2 in, 2 out]
                      n2488 = Fract/Exp String To Number(string=w3303) -> (number=w3306:dbl)  [unwired: 3 in, 1 out]
                      n2489 = Build Array (concatenate)(w3310, w3306) -> (w3309:dbl[])
                    }
                  }
                  n2490 = property on="data" class="Arr (strict)"("Value"=w3296) -> ()  [unwired: 2 in, 2 out]
                }
                frame #30 {
                  # "check if 1st channel \non Keithley 2182A 3\nis to be measured"
                  n2491 = property on="data" class="Arr (strict)"() -> ("Value"=w3312:dbl[])  [unwired: 2 in, 2 out]
                  n2492 = local read "2182A 3 ch1"() -> (w3311:bool)
                  n2493 = case shown="True" w3311 {
                    tunnel: w3312 -> [w3314 w3323]
                    tunnel: [w3314 w3322] -> w3313
                    frame False {
                      # "we are not measuring 2182A 3 channel 1 (2182A_3_ch1)"
                    }
                    frame True {
                      # "we are  measuring 2182A 3 channel 1 (2182A_3_ch1)"
                      n2494 = local read "2182A 3 addr"() -> (w3317:u8)
                      n2495 = Number To Decimal String(number=w3317) -> (decimal integer string=w3316:string)  [unwired: 1 in]
                      n2496 = GPIB Write(0:w3316, 1:":SENSe:DATA:FRES?") -> (6:w3321:errorcluster)  [unwired: 3 in, 1 out]
                      n2497 = GPIB Read(0:w3316, 1:200, 3:w3321) -> (5:w3315:string)  [unwired: 2 in, 2 out]
                      n2498 = Fract/Exp String To Number(string=w3315) -> (number=w3319:dbl)  [unwired: 3 in, 1 out]
                      n2499 = Build Array (concatenate)(w3323, w3319) -> (w3322:dbl[])
                    }
                  }
                  n2500 = property on="data" class="Arr (strict)"("Value"=w3313) -> ()  [unwired: 2 in, 2 out]
                }
                frame #31 {
                  # "check if 2nd channel \non Keithley 2182A 3\nis to be measured"
                  n2501 = property on="data" class="Arr (strict)"() -> ("Value"=w3325:dbl[])  [unwired: 2 in, 2 out]
                  n2502 = local read "2182A 3 ch2"() -> (w3324:bool)
                  n2503 = case shown="True" w3324 {
                    tunnel: w3325 -> [w3327 w3340]
                    tunnel: [w3327 w3339] -> w3326
                    frame False {
                      # "we are not measuring 2182A 3 channel 2 (2182A_3_ch2)"
                    }
                    frame True {
                      # "switching to channel 2 and then\nback to channel 1"
                      # "we are  measuring 2182A 3 channel 2 (2182A_3_ch2)"
                      n2504 = local read "2182A 3 addr"() -> (w3334:u8)
                      n2505 = Number To Decimal String(number=w3334) -> (decimal integer string=w3329:string)  [unwired: 1 in]
                      n2506 = GPIB Write(0:w3329, 1:":SENSe:CHAN 2") -> (6:w3331:errorcluster)  [unwired: 3 in, 1 out]
                      n2507 = GPIB Write(0:w3329, 1:":SENSe:DATA:FRES?", 3:w3331) -> (6:w3338:errorcluster)  [unwired: 2 in, 1 out]
                      n2508 = GPIB Read(0:w3329, 1:200, 3:w3338) -> (5:w3333:string, 7:w3330:errorcluster)  [unwired: 2 in, 1 out]
                      n2509 = GPIB Write(0:w3329, 1:":SENSe:CHAN 1", 3:w3330) -> ()  [unwired: 2 in, 2 out]
                      n2510 = Fract/Exp String To Number(string=w3333) -> (number=w3336:dbl)  [unwired: 3 in, 1 out]
                      n2511 = Build Array (concatenate)(w3340, w3336) -> (w3339:dbl[])
                    }
                  }
                  n2512 = property on="data" class="Arr (strict)"("Value"=w3326) -> ()  [unwired: 2 in, 2 out]
                }
                frame #32 {
                  # "check if 1st channel \non Keithley 2182A 4\nis to be measured"
                  n2513 = property on="data" class="Arr (strict)"() -> ("Value"=w3342:dbl[])  [unwired: 2 in, 2 out]
                  n2514 = local read "2182A 4 ch1"() -> (w3341:bool)
                  n2515 = case shown="True" w3341 {
                    tunnel: w3342 -> [w3344 w3353]
                    tunnel: [w3344 w3352] -> w3343
                    frame False {
                      # "we are not measuring 2182A 4 channel 1 (2182A_4_ch1)"
                    }
                    frame True {
                      # "we are  measuring 2182A 4 channel 1 (2182A_4_ch1)"
                      n2516 = local read "2182A 4 addr"() -> (w3347:u8)
                      n2517 = Number To Decimal String(number=w3347) -> (decimal integer string=w3346:string)  [unwired: 1 in]
                      n2518 = GPIB Write(0:w3346, 1:":SENSe:DATA:FRES?") -> (6:w3351:errorcluster)  [unwired: 3 in, 1 out]
                      n2519 = GPIB Read(0:w3346, 1:200, 3:w3351) -> (5:w3345:string)  [unwired: 2 in, 2 out]
                      n2520 = Fract/Exp String To Number(string=w3345) -> (number=w3349:dbl)  [unwired: 3 in, 1 out]
                      n2521 = Build Array (concatenate)(w3353, w3349) -> (w3352:dbl[])
                    }
                  }
                  n2522 = property on="data" class="Arr (strict)"("Value"=w3343) -> ()  [unwired: 2 in, 2 out]
                }
                frame #33 {
                  # "check if 2nd channel \non Keithley 2182A 4\nis to be measured"
                  n2523 = property on="data" class="Arr (strict)"() -> ("Value"=w3355:dbl[])  [unwired: 2 in, 2 out]
                  n2524 = local read "2182A 4 ch2"() -> (w3354:bool)
